vi "Reliability System MAIN (RT).vi"() -> ()   [LabVIEW 2013]
uses:
  TCP/PC/Event Mode.ctl
  RT subVIs/Controls/Stream RT FIFO Mode.ctl
  TCP/RT/RTsend PCrecv CMD.ctl
  <vilib>/FPGAPlugInAG/sbRIO-9626/niLvFpga_Open_sbRIO-9626.vi
  <vilib>/rvi/interface/common/dynamic/niFpgaDynamicAddResources.vi
  <vilib>/rvi/interface/common/niFpgaWaitOnOcc.vi
  <vilib>/Utility/error.llb/Error Cluster From Error Code.vi
  <vilib>/rvi/errors/niLvFpgaAdjustHostInterfaceError.vi
  <vilib>/Utility/file.llb/Read From Spreadsheet File (string).vi
  <vilib>/FPGAPlugInAG/Dynamic/niLvFpga_Reset_Dynamic.vi
  <vilib>/FPGAPlugInAG/Dynamic/niLvFpga_Run_Dynamic.vi
  <vilib>/rvi/interface/nirviOpenFPGA/nirviOpenFPGA.xnode
  FPGA Bitfiles/Reliability System.lvbitx
  FPGA/Reliability System (FPGA).vi
  <vilib>/rvi/interface/nirviMethod/nirviMethod.xnode
  <vilib>/rvi/interface/nirviReadWriteControl/nirviReadWriteControl.xnode
  <vilib>/NI_Real-Time Target Support.lvlib
  <vilib>/rvi/interface/Simulation/niFpgaSimulationCallBeginRW.vi
  NiFpgaLv.dll
  <vilib>/FPGAPlugInAG/Dynamic/niLvFpga_ReadFifo_Dynamic.vi
  <vilib>/rvi/errors/niLvFpgaMergeErrorWithErrorCode.vi
panel:
  out "Stream Error":i32
  out "FPGA Error":i32
  out "Sweeps Running":bool
  out "Sweep Count":i16
  out "Start  Ht Cmd":sgl
  out "End Ht Cmd":sgl
  out "Total Samples":sgl
  out "Start Sweep":bool
  out "Manual Cmd":bool
  out "Position Command Out":dbl
  out "Digital Output 4":bool
  out "Digital Output 3":bool
  out "Digital Output 2":bool
  out "Digital Output 1":bool
  out "Spare Output":dbl
  out "Power Supply Command":dbl
  out "Position Command":dbl
  in  "AI Loop Control (us)":u32
  in  "10kHz Loop Control (us)":u32
  in  "Stream Stop":bool
  out "RMC/DI7":bool
  out "RMC/DI6":bool
  out "RMC/DI5":bool
  out "RMC/DI4":bool
  out "AI Loop Time (us)":u32
  out "10kHz Loop Time (us)":u32
  out "Total (%)":dbl
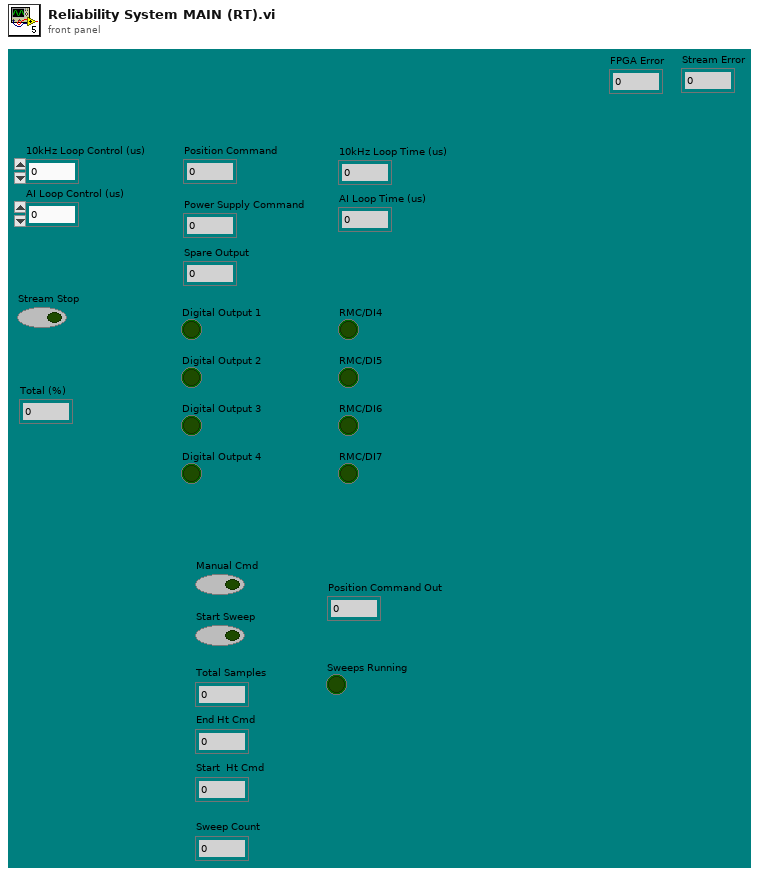
[diagram p1: front panel]
types:
  T1 = typedef "Event Mode.ctl" = enum16{"Init", "Get", "Set", "Destroy"}
  T2 = cluster{"DI Read Rate (sec)":dbl, "DI Read Timer":dbl, "Digital Outputs":bool[], "Analog Outputs":dbl[], "Sweeps Running":bool, "Sweep Parameters":sgl[], "Start Sweep":bool, "Manual Cmd":bool, "Startup Safety":bool, "Cal Cluster":cluster{"Slope":dbl[], "Offset":dbl[]}, "Cal Info":cluster{"Gauge#":i32, "CalDueDate":string}}
  T3 = enum16{"open", "replace", "create", "open or create", "replace or create", "replace or create with confirmation"}
  T4 = typedef "RTsend PCrecv CMD.ctl" = enum16{"Digital Inputs", "Connected?", "Data", "Data 2", "Cal2PC"}
  T5 = typedef "PCsend RTrecv CMD.ctl" = enum16{"ConnSettings", "Connect", "Stop", "Digital Outputs", "Analog Outputs", "Sweep Parameters", "Start Sweep", "Cal2RT", "Save Cal", "Load Cal"}
  T6 = cluster{"Slope":dbl[], "Offset":dbl[], "Gauge#":i32, "CalDueDate":string}
  T7 = cluster{"Sweeps Running":bool, dbl, "Current Sweep":i16}
  T8 = typedef "Stream RT FIFO Mode.ctl" = enum16{"Create", "Write", "Read", "Delete"}
  T9 = typedef "NI_Real-Time Target Support.lvlib/RT CPU Load.ctl" = cluster{"Total (%)":dbl, "Time Critical (%)":dbl, "Timed Structures (%)":dbl, "High (%)":dbl, "Above Normal (%)":dbl, "Normal (%)":dbl, "Background (%)":dbl, "Idle (%)":dbl, "ISR (%)":dbl}
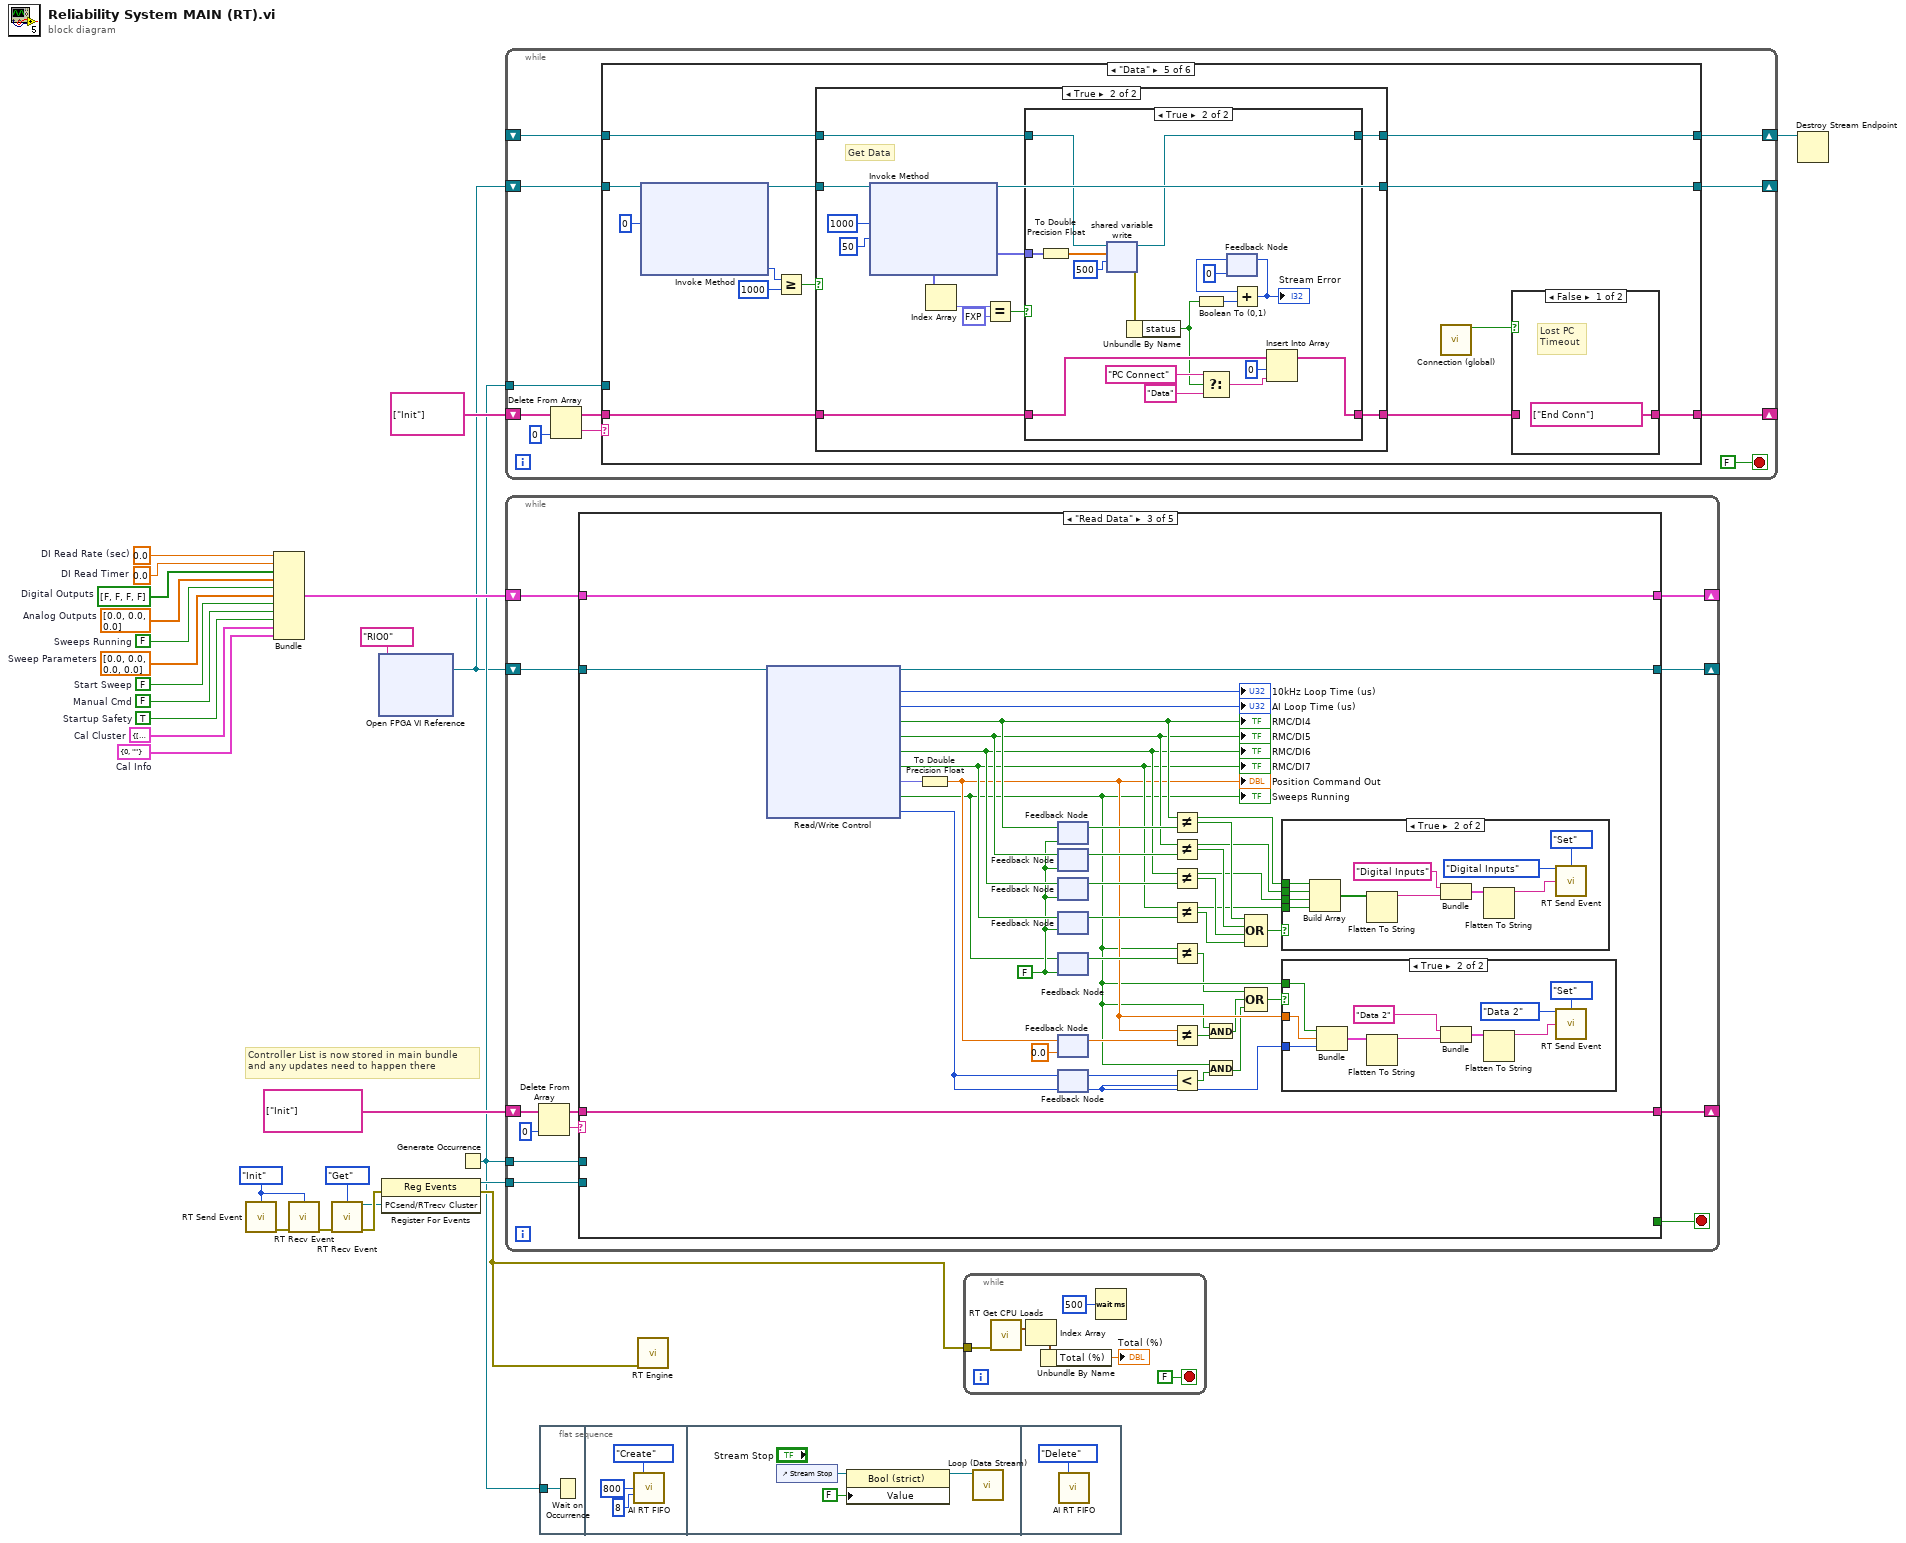
[diagram p0: block diagram]
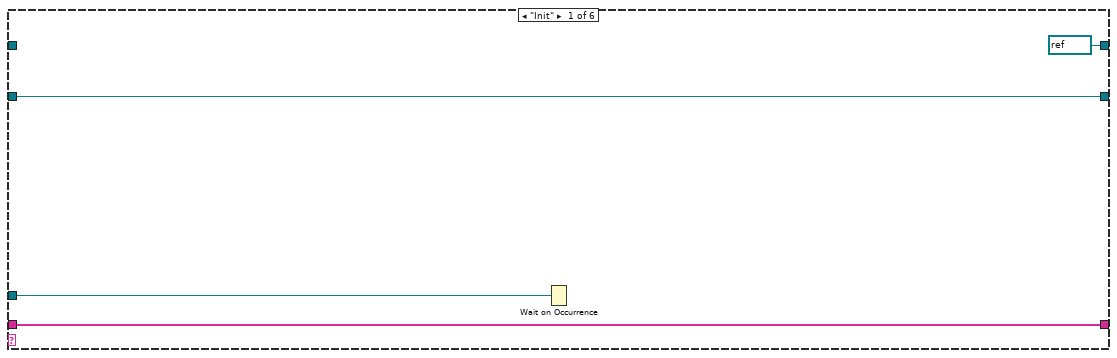
[diagram p2: hidden frame]
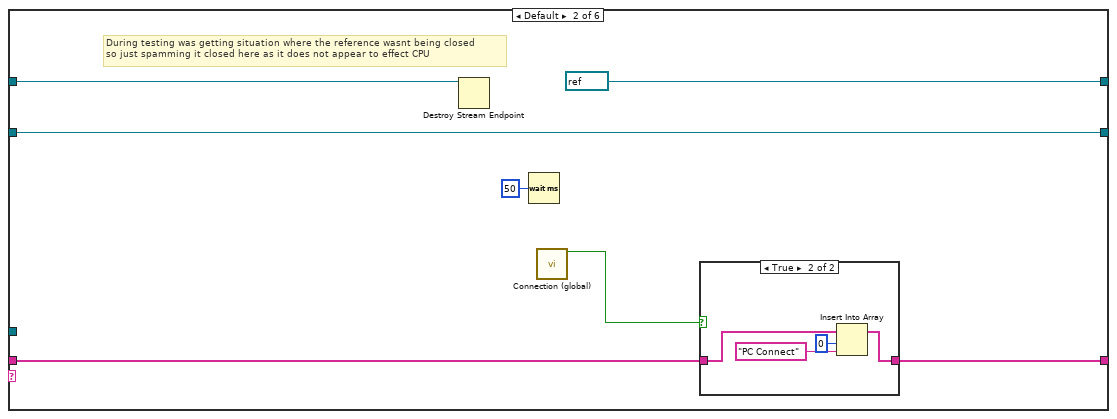
[diagram p3: hidden frame]
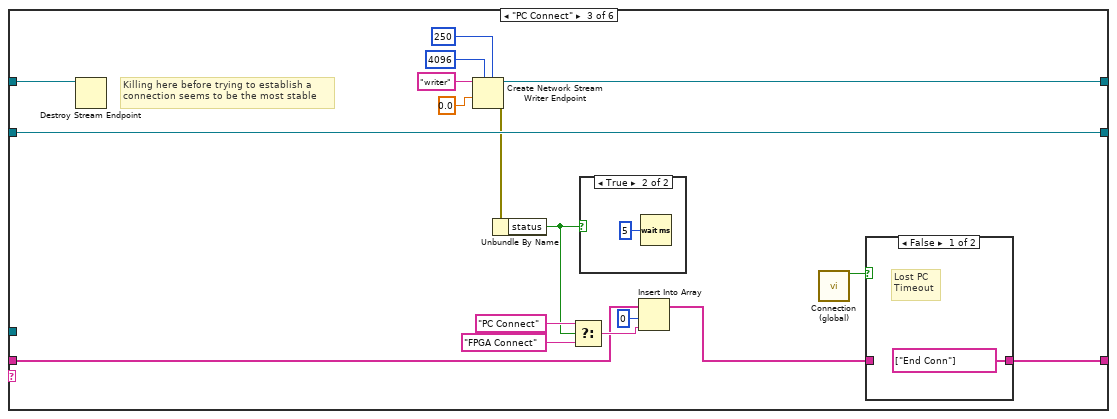
[diagram p5: hidden frame]
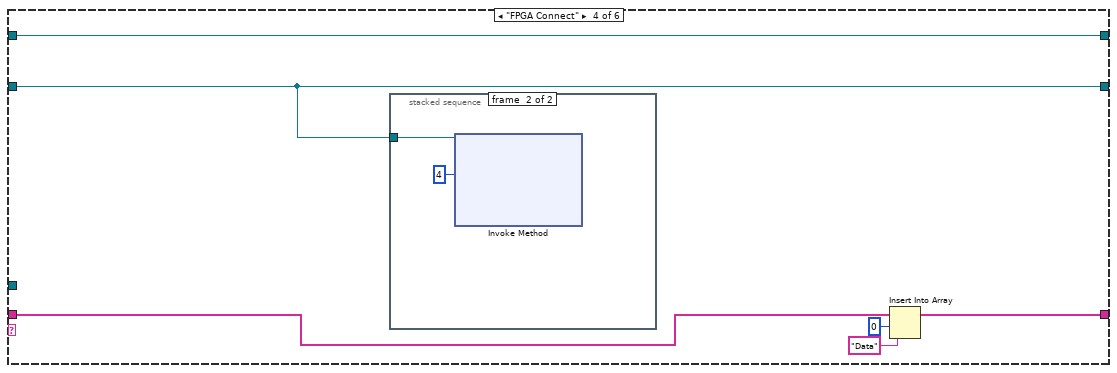
[diagram p8: hidden frame]
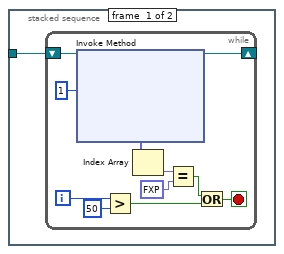
[diagram p9: hidden frame]
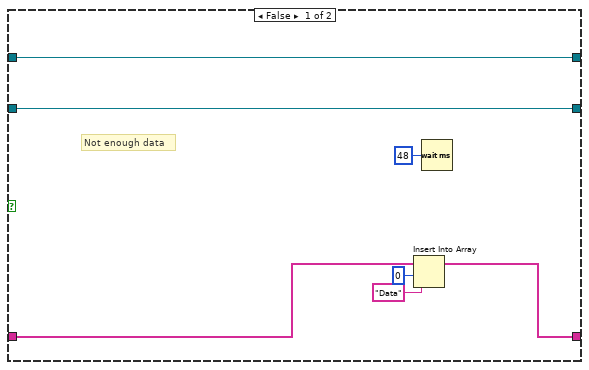
[diagram p11: hidden frame]
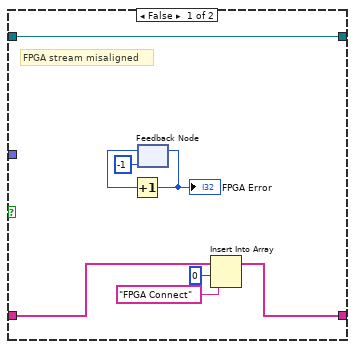
[diagram p12: hidden frame]
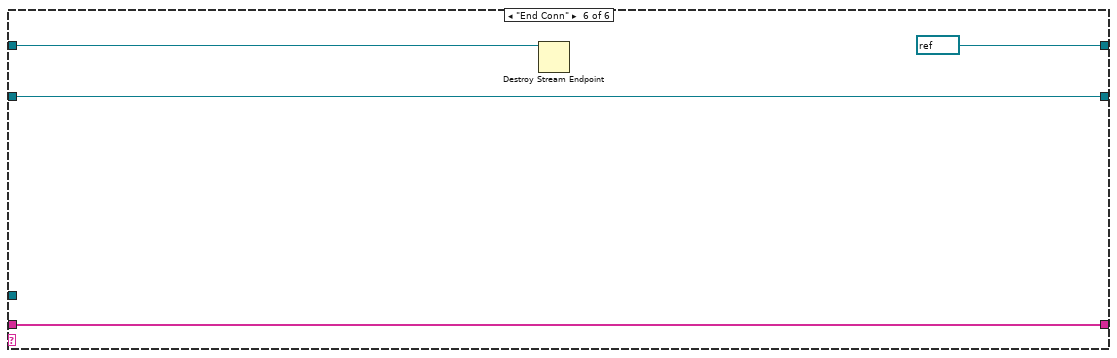
[diagram p13: hidden frame]
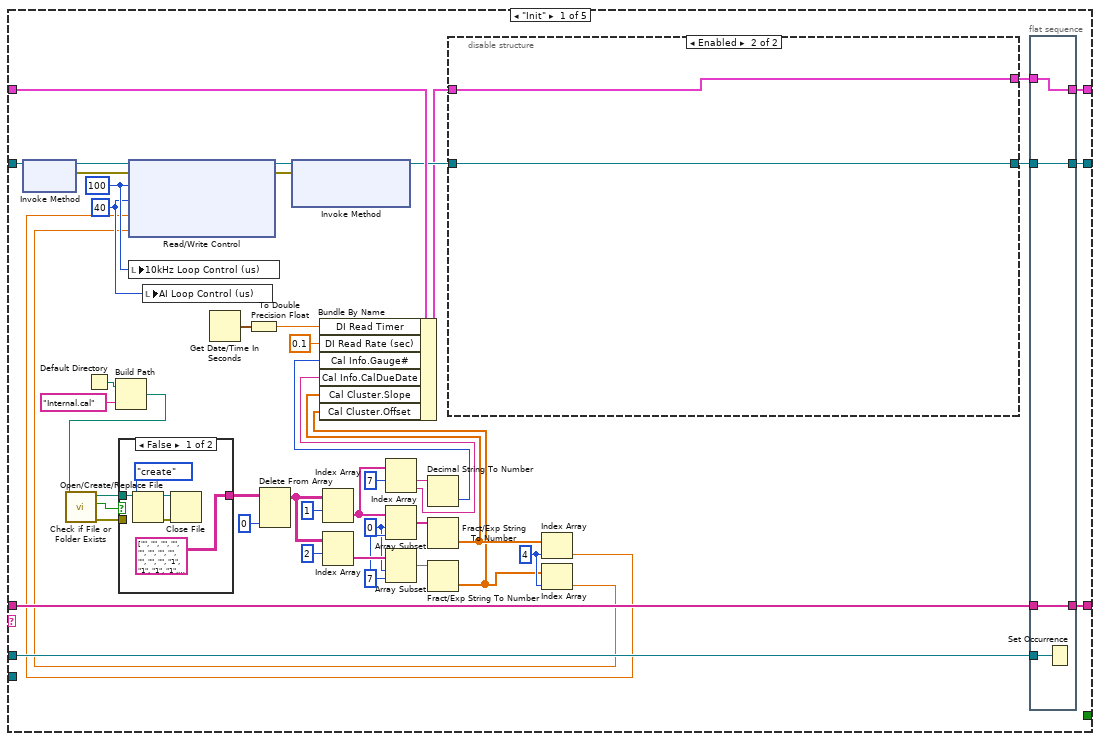
[diagram p14: hidden frame]
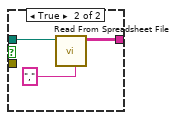
[diagram p15: hidden frame]
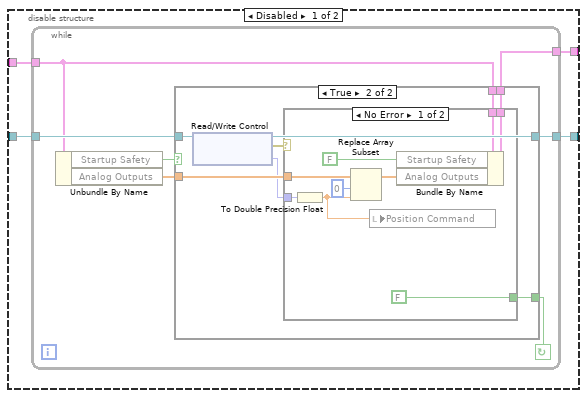
[diagram p16: hidden frame]
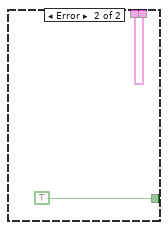
[diagram p18: hidden frame]
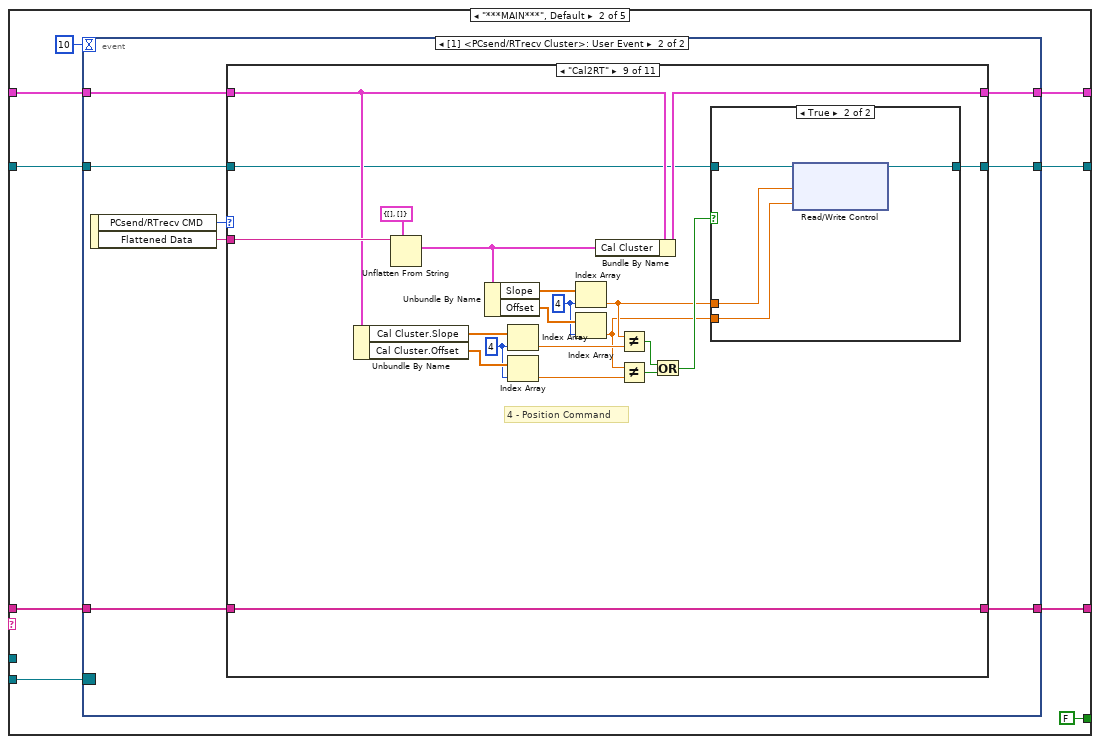
[diagram p19: hidden frame]
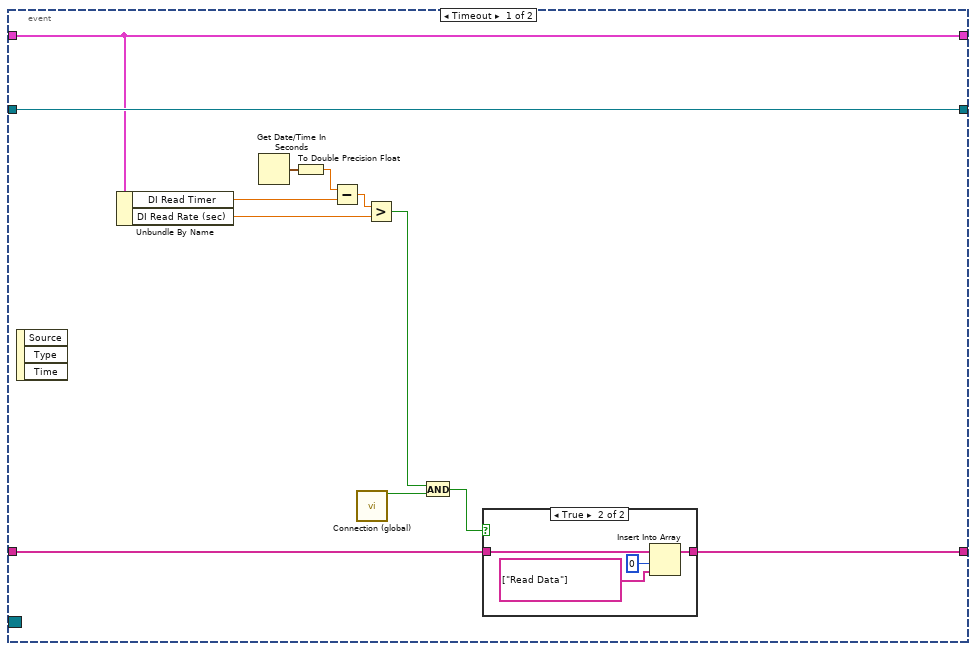
[diagram p20: hidden frame]
diagram:
  w3 = cluster{"Gauge#":i32, "CalDueDate":string} {"Gauge#"=0, "CalDueDate"=""}  # Cal Info
  w4 = cluster{"Slope":dbl[], "Offset":dbl[]} {"Slope"=[1.0, 1.0, 1.0, 1.0, 1.0, 1.0, 1.0], "Offset"=[0.0, 0.0, 0.0, 0.0, 0.0, 0.0, 0.0]}  # Cal Cluster
  w5 = TRUE  # Startup Safety
  w6 = FALSE  # Manual Cmd
  w7 = FALSE  # Start Sweep
  w8 = sgl[] [0.0, 0.0, 0.0, 0.0]  # Sweep Parameters
  w9 = FALSE  # Sweeps Running
  w12 = dbl[] [0.0, 0.0, 0.0]  # Analog Outputs
  w13 = bool[] [FALSE, FALSE, FALSE, FALSE]  # Digital Outputs
  w17 = 0.0  # DI Read Timer
  w18 = 0.0  # DI Read Rate (sec)
  w19 = Event_Mode."Init" ("Mode")
  # "Controller List is now stored in main bundle\nand any updates need to happen there"
  n1 = call "RT Send Event.vi"("Mode"=w19) -> ("Error Out"=w25:errorcluster)  [unwired: 13 in, 1 out]
  n2 = Bundle("DI Read Rate (sec)"=w18, "DI Read Timer"=w17, "Digital Outputs"=w13, "Analog Outputs"=w12, "Sweeps Running"=w9, "Sweep Parameters"=w8, "Start Sweep"=w7, "Manual Cmd"=w6, "Startup Safety"=w5, "Cal Cluster"=w4, "Cal Info"=w3) -> (w26:T2)  [unwired: 1 in]
  n3 = call "RT Recv Event.vi"("Mode"=w19, "Error In"=w25) -> ("Error Out"=w24:errorcluster)  [unwired: 12 in, 1 out]
  n4 = call "RT Recv Event.vi"("Mode"=Event_Mode."Get", "Error In"=w24) -> ("PCsend/RTrecv Cluster"=w22:refnum<user-event>, "Error Out"=w23:errorcluster)  [unwired: 12 in]
  n5 = xnode ("Open FPGA VI Reference")("resource name"=tag "RIO0") -> ("FPGA VI Reference Out"=w1:refnum<k20>)  [unwired: 1 in, 1 out]
  n6 = register-events(error in=w23, w22) -> (reference out=w21:refnum<event-registration>, error out=w16:errorcluster)  [unwired: 1 in]
  n7 = Generate Occurrence() -> (w10:refnum<k4>)
  n8 = while {
    shift-right: [w32] -> _
    shift-left: string[] ["Init"] -> [w36]
    tunnel: w10 -> [w31]
    shift-right: [w30] -> w2
    shift-left: _ -> [w29]
    shift-right: [w27] -> _
    shift-left: w1 -> [w28]
    stop <- FALSE stop-if-true
    n9 = Delete From Array(array=w36, index=0) -> (deleted portion=w34:string, array with subset deleted=w33:string[])  [unwired: 1 in]
    n10 = case shown="\"Data\"" w34 {
      tunnel: w33 -> [w40 w45 w64 w76 w97 w156]
      tunnel: [w40 w44 w57 w75 w95 w156] -> w32
      tunnel: w31 -> [w41 _ _ _ _ _]
      tunnel: [refnum<k21> refnum ("writer name") refnum<k21> refnum ("writer name") w55 w79 w98 refnum<k21> refnum ("writer name")] -> w30
      tunnel: w29 -> [_ w43 w54 w79 w99 w154]
      tunnel: w28 -> [w38 w48 w61 w78 w105 w155]
      tunnel: [w38 w48 w61 w78 w100 w155] -> w27
      frame "Init" {
        n11 = Wait on Occurrence(2:w41) -> ()  [unwired: 2 in, 1 out]
      }
      frame Default {
        # "During testing was getting situation where the reference wasnt being closed\nso just spamming it closed here as it does not appear to effect CPU"
        n12 = Destroy Stream Endpoint(11:w43) -> ()  [unwired: 1 in, 1 out]
        n13 = Wait (ms)(milliseconds to wait=u32 50) -> ()  [unwired: 1 out]
        n14 = call "Connection (global).vi"() -> ("PC Connected Out"=w46:bool)  [unwired: 15 in]
        n15 = case shown="True" w46 {
          tunnel: w45 -> [w49 w53]
          tunnel: [w49 w52] -> w44
          frame False {
          }
          frame True {
            n16 = Insert Into Array(array=w53, index=0, new element="PC Connect" ("new element/subarray")) -> (w52:string[])
          }
        }
      }
      frame "PC Connect" {
        # "Killing here before trying to establish a\nconnection seems to be the most stable"
        n17 = Destroy Stream Endpoint(11:w54) -> ()  [unwired: 1 in, 1 out]
        n18 = Create Network Stream Writer Endpoint(5:250 ("timeout in ms (-1)"), 7:4096 ("writer buffer size"), 9:0.0, 11:"writer" ("writer name")) -> (0:w56:errorcluster, 3:w55:refnum<k21>)  [unwired: 3 in]
        n19 = Unbundle By Name(w56) -> ("status"=w60:bool)
        n20 = Select(t="PC Connect" ("writer name"), s=w60, f="FPGA Connect" ("writer name")) -> (s? t:f=w66:string)
        n21 = case shown="True" w60 {
          frame False {
          }
          frame True {
            n22 = Wait (ms)(milliseconds to wait=u32 5) -> ()  [unwired: 1 out]
          }
        }
        n23 = Insert Into Array(array=w64, index=0, new element=w66) -> (w58:string[])
        n24 = call "Connection (global).vi"() -> ("PC Connected Out"=w59:bool)  [unwired: 15 in]
        n25 = case shown="False" w59 {
          tunnel: w58 -> [_ w72]
          tunnel: [string[] ["End Conn"] w72] -> w57
          frame False {
            # "Lost PC\nTimeout"
          }
          frame True {
            # "Still have PC\nContinue"
          }
        }
      }
      frame "FPGA Connect" {
        n26 = stacked-sequence {
          tunnel: w78 -> [w80 w93]
          frame #0 {
            n27 = while {
              shift-right: [w90] -> _
              shift-left: w80 -> [w91]
              i -> [w85]
              stop <- w82 stop-if-true
              n28 = xnode "Invoke Method"("FPGA VI Reference In"=w91, "Number of Elements"=u32 1) -> ("FPGA VI Reference Out"=w90:refnum<k20>, "Data"=w87:fxp<+/-,24,5>[])  [unwired: 2 in, 2 out]
              n29 = Greater?(x=w85, y=50) -> (0:w84:bool)
              n30 = Index Array(array=w87) -> (element=w86:fxp<+/-,24,5>)  [unwired: 1 in]
              n31 = Equal?(x=w86, y=fxp<+/-,24,5> -15.0) -> (x = y?=w83:bool)
              n32 = Or(x=w83, y=w84) -> (x .or. y?=w82:bool)
            }
          }
          frame #1 {
            n33 = xnode "Invoke Method"("FPGA VI Reference In"=w93, "Number of Elements"=u32 4) -> ()  [unwired: 2 in, 4 out]
          }
        }
        n34 = Insert Into Array(array=w76, index=0, new element="Data" ("new element/subarray")) -> (w75:string[])
      }
      frame "Data" {
        n35 = xnode "Invoke Method"("FPGA VI Reference In"=w105, "Number of Elements"=u32 0) -> ("FPGA VI Reference Out"=w101:refnum<k20>, "Elements Remaining"=w104:u32)  [unwired: 2 in, 2 out]
        n36 = Greater Or Equal?(x=w104, y=u32 1000) -> (x >= y?=w102:bool)
        n37 = case shown="True" w102 {
          tunnel: w101 -> [w114 w127]
          tunnel: [w114 w126] -> w100
          tunnel: w99 -> [w113 w120]
          tunnel: [w113 w119] -> w98
          tunnel: w97 -> [w112 w118]
          tunnel: [w111 w117] -> w96
          frame False {
            # "Not enough data"
            n38 = Insert Into Array(array=w112, index=0, new element="Data" ("new element/subarray")) -> (w111:string[])
            n39 = Wait (ms)(milliseconds to wait=u32 48) -> ()  [unwired: 1 out]
          }
          frame True {
            # "Get Data"
            n40 = xnode "Invoke Method"("FPGA VI Reference In"=w127, "Number of Elements"=u32 1000 ("y"), "Timeout (ms)"=50) -> ("FPGA VI Reference Out"=w126:refnum<k20>, "Data"=w116:fxp<+/-,24,5>[])  [unwired: 1 in, 2 out]
            n41 = Index Array(array=w116) -> (element=w122:fxp<+/-,24,5>)  [unwired: 1 in]
            n42 = Equal?(x=w122, y=fxp<+/-,24,5> -15.0) -> (x = y?=w121:bool)
            n43 = case shown="True" w121 {
              tunnel: w120 -> [w135 w151]
              tunnel: [w135 w150] -> w119
              tunnel: w118 -> [w134 w148]
              tunnel: [w131 w147] -> w117
              tunnel: w116 -> [_ w149]
              frame False {
                # "FPGA stream misaligned"
                n44 = feedback #1(-1) -> (w129:i32)
                n45 = Increment(x=w129) -> (x+1=w128:i32)
                "FPGA Error" <- w128
                n46 = feedback-in #1(w128) -> ()
                n47 = Insert Into Array(array=w134, index=0, new element="FPGA Connect" ("new element/subarray")) -> (w131:string[])
              }
              frame True {
                n48 = To Double Precision Float(number=w149) -> (double precision float=w141:dbl[])
                n49 = shared-variable-write(w151, w141, 500 ("timeout ms (-1)")) -> (w150:refnum<k21>, w145:errorcluster)  [unwired: 1 in, 1 out]
                n50 = Unbundle By Name(w145) -> ("status"=w136:bool)
                n51 = Boolean To (0,1)(Boolean=w136) -> (0, 1=w137:i16)
                n52 = Select(t="PC Connect", s=w136, f="Data") -> (s? t:f=w142:string)
                n53 = feedback #2(0) -> (w139:i32)
                n54 = Add(x=w139, y=w137) -> (x+y=w138:i32)
                "Stream Error" <- w138
                n55 = feedback-in #2(w138) -> ()
                n56 = Insert Into Array(array=w148, index=0, new element=w142) -> (w147:string[])
              }
            }
          }
        }
        n57 = call "Connection (global).vi"() -> ("PC Connected Out"=w94:bool)  [unwired: 15 in]
        n58 = case shown="False" w94 {
          tunnel: w96 -> [_ w108]
          tunnel: [string[] ["End Conn"] w108] -> w95
          frame False {
            # "Lost PC\nTimeout"
          }
          frame True {
            # "Still have PC\nContinue"
          }
        }
      }
      frame "End Conn" {
        n59 = Destroy Stream Endpoint(11:w154) -> ()  [unwired: 1 in, 1 out]
      }
    }
  }
  n60 = while {
    shift-right: [w164] -> _
    shift-left: string[] ["Init"] -> [w168]
    shift-right: [w161] -> _
    shift-left: w26 -> [w163]
    shift-right: [w159] -> _
    shift-left: w1 -> [w160]
    tunnel: w21 -> [w158]
    tunnel: w10 -> [w157]
    stop <- w162 stop-if-true
    n61 = Delete From Array(array=w168, index=0) -> (deleted portion=w165:string, array with subset deleted=w166:string[])  [unwired: 1 in]
    n62 = case shown="\"Read Data\"" w165 {
      tunnel: w166 -> [w211 w270 w476 w523 w590]
      tunnel: [w210 w266 w476 w523 w589] -> w164
      tunnel: w163 -> [w207 w269 w459 w503 w595]
      tunnel: [_ FALSE _ _ _] -> w162
      tunnel: [w196 w267 w459 w502 w594] -> w161
      tunnel: w160 -> [w213 w264 w477 w505 w597]
      tunnel: [w212 w263 w475 w522 w597] -> w159
      tunnel: w158 -> [_ w262 _ _ _]
      tunnel: w157 -> [w209 _ _ _ _]
      frame "Init" {
        w173 = 4 ("index")
        w187 = 7 ("length")
        w186 = 0 ("index")
        w178 = u32 40 ("100kHz Loop Control (us)")
        w201 = u32 100 ("10kHz Loop Control (us)")
        n63 = xnode "Invoke Method"("FPGA VI Reference In"=w213) -> ("FPGA VI Reference Out"=w206:refnum<k20>, "error out"=w205:errorcluster)  [unwired: 1 in]
        n64 = Default Directory() -> (w176:path)
        n65 = Build Path(base path=w176, name or relative path="Internal.cal") -> (appended path=w174:path)
        n66 = call <vilib>:"Check if File or Folder Exists.vi"("path"=w174) -> ("error out"=w177:errorcluster, "file or folder exists?"=w194:bool, "dup path"=w195:path)  [unwired: 8 in]
        n67 = case shown="False" w194 {
          tunnel: [string[][] [["", "", "", "", "", "", "", "", "", ""], ["", "1", "1", "1", "1", "1", "1", "1", "1234", "01/01/00"], ["", "0", "0", "0", "0", "0", "0", "0", "0", "0"]] ("all rows") w222] -> w185
          tunnel: w195 -> [w219 w220]
          tunnel: w177 -> [_ _]
          frame False {
            n68 = Open/Create/Replace File(file path (use dialog)=w219, operation (0:open)=T3."create") -> (refnum out=w218:refnum<file>, error out=w217:errorcluster)  [unwired: 4 in, 1 out]
            n69 = Close File(refnum=w218, error in=w217) -> ()  [unwired: 2 out]
          }
          frame True {
            n70 = call-poly <vilib>:"Read From Spreadsheet File.vi"("delimiter (\\t)"="," ("delimiter (\\t)"), "file path (dialog if empty)"=w220) -> ("all rows"=w222:string[][])  [unwired: 5 in, 4 out]
          }
        }
        n71 = local write "10kHz Loop Control (us)"(w201) -> ()
        n72 = local write "AI Loop Control (us)"(w178) -> ()
        n73 = Get Date/Time In Seconds() -> (seconds since 1Jan1904=w214:timestamp)
        n74 = To Double Precision Float(number=w214) -> (double precision float=w208:dbl)
        n75 = Delete From Array(array=w185, index (col)=0 ("disabled index (col)")) -> (array with subset deleted=w183:string[][])  [unwired: 2 in, 1 out]
        n76 = Index Array(array=w183, index (row)=1) -> (element=w191:string[])  [unwired: 1 in]
        n77 = Index Array(array=w183, index (row)=2) -> (element=w188:string[])  [unwired: 1 in]
        n78 = Index Array(array=w191, index #1=7 ("index")) -> (element #1=w193:string, element #2=w179:string)  [unwired: 1 in]
        n79 = Array Subset(array=w191, index=w186, length=w187) -> (w189:string[])
        n80 = Array Subset(array=w188, index=w186, length=w187) -> (w190:string[])
        n81 = Decimal String To Number(string=w193) -> (number=w180:i32)  [unwired: 2 in, 1 out]
        n82 = Fract/Exp String To Number(string=w189) -> (number=w172:dbl[])  [unwired: 3 in, 1 out]
        n83 = Fract/Exp String To Number(string=w190) -> (number=w171:dbl[])  [unwired: 3 in, 1 out]
        n84 = Bundle By Name(cluster=w207, "DI Read Timer"=w208, "DI Read Rate (sec)"=0.1, "Cal Info.Gauge#"=w180, "Cal Info.CalDueDate"=w179, "Cal Cluster.Slope"=w172, "Cal Cluster.Offset"=w171) -> (w198:T2)
        n85 = Index Array(array=w172, index=w173) -> (element=w170:dbl)
        n86 = Index Array(array=w171, index=w173) -> (element=w169:dbl)
        n87 = xnode "Read/Write Control"("FPGA VI Reference In"=w206, "error in"=w205, "10kHz Loop Control (us)"=w201, "AI Loop Control (us)"=w178, "Ht Cmd Slope"=w170, "Ht Cmd Offset"=w169) -> ("FPGA VI Reference Out"=w203:refnum<k20>, "error out"=w204:errorcluster)
        n88 = xnode "Invoke Method"("FPGA VI Reference In"=w203, "error in"=w204) -> ("FPGA VI Reference Out"=w200:refnum<k20>)  [unwired: 1 in, 1 out]
        n89 = disable-structure shown="Enabled" {
          disable-tunnel: w200 -> [w226 w256]
          disable-tunnel: [w225 w256] -> w199
          disable-tunnel: w198 -> [w224 w257]
          disable-tunnel: [w223 w257] -> w197
          frame Disabled {
            n90 = while {
              tunnel: w226 -> [w231]
              tunnel: [w230] -> w225
              tunnel: w224 -> [w229]
              tunnel: [w228] -> w223
              stop <- w227 continue-if-true
              n91 = Unbundle By Name(w229) -> ("Startup Safety"=w233:bool, "Analog Outputs"=w232:dbl[])
              n92 = case shown="True" w233 {
                selector: w233 -> [w234 _]
                tunnel: w231 -> [w236 w244]
                tunnel: [w236 w243] -> w230
                tunnel: [w235 w241] -> w228
                tunnel: w229 -> [w235 w240]
                tunnel: w232 -> [_ w239]
                tunnel: [w234 w237] -> w227
                frame False {
                }
                frame True {
                  n93 = xnode "Read/Write Control"("FPGA VI Reference In"=w244) -> ("FPGA VI Reference Out"=w243:refnum<k20>, "error out"=w242:errorcluster, "Height Raw"=w238:fxp<+/-,24,5>)  [unwired: 1 in]
                  n94 = case shown="No Error" w242 {
                    tunnel: [w253 w255] -> w241
                    tunnel: w240 -> [w252 w255]
                    tunnel: w239 -> [w251 _]
                    tunnel: w238 -> [w248 _]
                    tunnel: [FALSE TRUE] -> w237
                    frame No Error {
                      n95 = To Double Precision Float(number=w248) -> (double precision float=w247:dbl)
                      n96 = Replace Array Subset(array=w251, new element=w247, index=0) -> (w250:dbl[])
                      n97 = local write "Position Command"(w247) -> ()
                      n98 = Bundle By Name(cluster=w252, "Startup Safety"=FALSE, "Analog Outputs"=w250) -> (w253:T2)
                    }
                    frame Error {
                    }
                  }
                }
              }
            }
          }
          frame Enabled {
          }
        }
        n99 = flat-sequence {
          tunnel: [w259] -> w212
          tunnel: w211 -> [w261]
          tunnel: [w261] -> w210
          tunnel: w209 -> [w260]
          tunnel: w199 -> [w259]
          tunnel: w197 -> [w258]
          tunnel: [w258] -> w196
          frame #0 {
            n100 = Set Occurrence(w260) -> ()
          }
        }
      }
      frame "***MAIN***", Default {
        n101 = event shown="[1] <PCsend/RTrecv Cluster>: User Event" {
          selector: w262 -> [_ _]
          dyn-events: _ -> [_ _]
          timeout: 10 -> [_ _]
          tunnel: w270 -> [w280 w292]
          tunnel: w269 -> [w274 w295]
          tunnel: [w274 w294] -> w267
          tunnel: [w275 w291] -> w266
          tunnel: w264 -> [w279 w288]
          tunnel: [w279 w290] -> w263
          event Timeout {
            n102 = event-data() -> ()  [unwired: 1 in, 3 out]
            n103 = Unbundle By Name(w274) -> ("DI Read Timer"=w282:dbl, "DI Read Rate (sec)"=w281:dbl)
            n104 = Get Date/Time In Seconds() -> (seconds since 1Jan1904=w278:timestamp)
            n105 = To Double Precision Float(number=w278) -> (double precision float=w276:dbl)
            n106 = Subtract(x=w276, y=w282) -> (x-y=w277:dbl)
            n107 = call "Connection (global).vi"() -> ("PC Connected Out"=w273:bool)  [unwired: 15 in]
            n108 = Greater?(x=w277, y=w281) -> (0:w272:bool)
            n109 = And(x=w272, y=w273) -> (x .and. y?=w271:bool)
            n110 = case shown="True" w271 {
              tunnel: w280 -> [w283 w287]
              tunnel: [w283 w286] -> w275
              frame False {
              }
              frame True {
                n111 = Insert Into Array(array=w287, index=0, new element=string[] ["Read Data"]) -> (w286:string[])
              }
            }
          }
          event User Event {
            n112 = event-data() -> ("PCsend/RTrecv CMD"=w289:T5, "Flattened Data"=w293:string)  [unwired: 1 in]
            n113 = case shown="\"Cal2RT\"" w289 {
              tunnel: w295 -> [w298 w300 w303 w306 w315 w328 w348 w365 w385 w427 w434]
              tunnel: [w298 w300 w303 w306 w314 w322 w347 w363 w386 w428 w434] -> w294
              tunnel: w293 -> [_ _ _ _ w321 w337 w350 w366 w387 w429 _]
              tunnel: w292 -> [w297 w299 w302 w305 w319 w333 w344 w360 w372 w426 w443]
              tunnel: [w297 w299 w302 w305 w318 w332 w344 w359 w372 w426 w443] -> w291
              tunnel: w288 -> [w296 w301 w304 w307 w313 w338 w346 w362 w370 w425 w442]
              tunnel: [w296 w301 w304 w307 w313 w338 w346 w362 w369 w425 w442] -> w290
              frame Default {
                # "Shouldn't ever get here\nwhich would mean something is not setup correctly"
              }
              frame "ConnSettings" {
              }
              frame "Connect" {
              }
              frame "Stop" {
              }
              frame "Digital Outputs" {
                n114 = Unflatten From String(type=bool[] [FALSE, FALSE, FALSE, FALSE], binary string=w321) -> (value=w312:bool[])  [unwired: 3 in, 2 out]
                n115 = Index Array(array=w312) -> (element #1=→"Digital Output 1":bool, element #2=→"Digital Output 2":bool, element #3=→"Digital Output 3":bool, element #4=→"Digital Output 4":bool)  [unwired: 4 in]
                n116 = Bundle By Name(cluster=w315, "Digital Outputs"=w312) -> (w314:T2)
                n117 = Insert Into Array(array=w319, index=0, new element="Write Outputs" ("new element/subarray")) -> (w318:string[])
              }
              frame "Analog Outputs" {
                n118 = Unflatten From String(type=dbl[] [0.0, 0.0, 0.0], binary string=w337) -> (value=w331:dbl[])  [unwired: 3 in, 2 out]
                n119 = Unbundle By Name(w328) -> ("Analog Outputs"=w327:dbl[])
                n120 = Index Array(array=w331) -> (element #1=w325:dbl, element #2=→"Power Supply Command":dbl, element #3=→"Spare Output":dbl)  [unwired: 3 in]
                "Position Command" <- w325
                n121 = Index Array(array=w327) -> (element=w326:dbl)  [unwired: 1 in]
                n122 = Bundle By Name(cluster=w328, "Analog Outputs"=w331) -> (w323:T2)
                n123 = Not Equal?(x=w326, y=w325) -> (x != y?=w324:bool)
                n124 = Insert Into Array(array=w333, index=0, new element="Write Outputs" ("new element/subarray")) -> (w332:string[])
                n125 = case shown="True" w324 {
                  tunnel: w323 -> [w339 w343]
                  tunnel: [w339 w341] -> w322
                  frame False {
                  }
                  frame True {
                    w340 = TRUE ("Manual Cmd")
                    n126 = local write "Manual Cmd"(w340) -> ()
                    n127 = Bundle By Name(cluster=w343, "Manual Cmd"=w340, "Start Sweep"=FALSE) -> (w341:T2)
                  }
                }
              }
              frame "Sweep Parameters" {
                n128 = Unflatten From String(type=sgl[] [0.0, 0.0, 0.0, 0.0], binary string=w350) -> (value=w345:sgl[])  [unwired: 3 in, 2 out]
                n129 = Index Array(array=w345) -> (element #1=→"Total Samples":sgl, element #2=→"End Ht Cmd":sgl, element #3=→"Start  Ht Cmd":sgl, element #4=w354:sgl)  [unwired: 4 in]
                n130 = To Word Integer(number=w354) -> (16bit integer=→"Sweep Count":i16)
                n131 = Bundle By Name(cluster=w348, "Sweep Parameters"=w345) -> (w347:T2)
              }
              frame "Start Sweep" {
                n132 = Unflatten From String(type=FALSE, binary string=w366) -> (value=w357:bool)  [unwired: 3 in, 2 out]
                "Start Sweep" <- w357
                n133 = Not(x=w357) -> (.not. x?=w356:bool)
                "Manual Cmd" <- w356
                n134 = Insert Into Array(array=w360, index=0, new element=string[] ["Write Outputs", "Handle Sweep Start"]) -> (w359:string[])
                n135 = Bundle By Name(cluster=w365, "Start Sweep"=w357, "Manual Cmd"=w356) -> (w363:T2)
              }
              frame "Cal2RT" {
                w378 = 4 ("index")
                w377 = 4 ("index")
                # "4 - Position Command"
                n136 = Unbundle By Name(w385) -> ("Cal Cluster.Slope"=w382:dbl[], "Cal Cluster.Offset"=w381:dbl[])
                n137 = Unflatten From String(type=cluster{"Slope":dbl[], "Offset":dbl[]} {"Slope"=[], "Offset"=[]}, binary string=w387) -> (value=w383:cluster{"Slope":dbl[], "Offset":dbl[]})  [unwired: 3 in, 2 out]
                n138 = Unbundle By Name(w383) -> ("Slope"=w380:dbl[], "Offset"=w379:dbl[])
                n139 = Index Array(array=w382, index=w377) -> (element=w376:dbl)
                n140 = Index Array(array=w381, index=w377) -> (element=w375:dbl)
                n141 = Index Array(array=w380, index=w378) -> (element=w368:dbl)
                n142 = Index Array(array=w379, index=w378) -> (element=w367:dbl)
                n143 = Bundle By Name(cluster=w385, "Cal Cluster"=w383) -> (w386:T2)
                n144 = Not Equal?(x=w368, y=w376) -> (x != y?=w374:bool)
                n145 = Not Equal?(x=w367, y=w375) -> (x != y?=w373:bool)
                n146 = Or(x=w374, y=w373) -> (x .or. y?=w371:bool)
                n147 = case shown="True" w371 {
                  tunnel: w370 -> [w388 w392]
                  tunnel: [w388 w391] -> w369
                  tunnel: w368 -> [_ w390]
                  tunnel: w367 -> [_ w389]
                  frame False {
                  }
                  frame True {
                    n148 = xnode "Read/Write Control"("FPGA VI Reference In"=w392, "Ht Cmd Slope"=w390, "Ht Cmd Offset"=w389) -> ("FPGA VI Reference Out"=w391:refnum<k20>)  [unwired: 1 in, 1 out]
                  }
                }
              }
              frame "Save Cal" {
                (unwired) path "c/Internal.cal"
                w402 = ""
                n149 = Unbundle By Name(w427) -> ("Cal Cluster.Slope"=w399:dbl[], "Cal Cluster.Offset"=w396:dbl[])
                n150 = Unflatten From String(type=cluster{"Gauge#":i32, "CalDueDate":string} {"Gauge#"=0, "CalDueDate"=""}, binary string=w429) -> (value=w400:cluster{"Gauge#":i32, "CalDueDate":string})  [unwired: 3 in, 2 out]
                n151 = Unbundle By Name(w400) -> ("Gauge#"=w398:i32, "CalDueDate"=w397:string)
                n152 = Default Directory() -> (w395:path)
                n153 = Number To Decimal String(number=w398) -> (decimal integer string=w401:string)  [unwired: 1 in]
                n154 = Number To Fractional String(number=w399) -> (F-format string=w406:string[])  [unwired: 3 in]
                n155 = Number To Fractional String(number=w396) -> (F-format string=w404:string[])  [unwired: 3 in]
                n156 = Build Path(base path=w395, name or relative path="Internal.cal") -> (appended path=w393:path)
                n157 = Build Array (concatenate)(w406, w401, w397) -> (w405:string[])
                n158 = Build Array (concatenate)(w404, w402, w402) -> (w403:string[])
                n159 = Replace Array Subset(array=string[][] [["Power Supply Voltage", "Level Sender Voltage", "AI-3 Spare", "Height Gauge", "Servo Motor Control", "Spare Analog Output 1", "Spare Analog Output 2", "Gauge Number", "CalDueDate"], ["", "", "", "", "", "", "", "", ""], ["", "", "", "", "", "", "", "", ""]], new element=w405, index (row)=1) -> (w414:string[][])  [unwired: 1 in]
                n160 = Bundle By Name(cluster=w427, "Cal Info"=w400) -> (w428:T2)
                n161 = Replace Array Subset(array=w414, new element=w403, index (row)=2) -> (w413:string[][])  [unwired: 1 in]
                n162 = Insert Into Array(array=w413, index (col)=0 ("disabled index (col)"), new element=string[] ["Channel Name", "Slope", "Offset"]) -> (w408:string[][])  [unwired: 1 in]
                n163 = Open/Create/Replace File(file path (use dialog)=w393, operation (0:open)=T3."open or create") -> (refnum out=w416:refnum<file>, error out=w415:errorcluster)  [unwired: 4 in, 1 out]
                n164 = Array To Spreadsheet String(delimiter (Tab)=",", array=w408, 3:"%s" ("format string")) -> (spreadsheet string=w418:string)
                n165 = Write to Text File(file (use dialog)=w416, text=w418, error in=w415) -> (refnum out=w422:refnum<file>, error out=w423:errorcluster)  [unwired: 1 in, 1 out]
                n166 = Close File(refnum=w422, error in=w423) -> (error out=w421:errorcluster)  [unwired: 1 out]
                n167 = call <vilib>:"Clear Errors.vi"("error in (no error)"=w421) -> ()  [unwired: 6 in, 1 out]
              }
              frame "Load Cal" {
                # "This is a request from the PC to be sent the cal file settings"
                n168 = Unbundle By Name(w434) -> ("Cal Cluster.Slope"=w433:dbl[], "Cal Cluster.Offset"=w432:dbl[], "Cal Info.Gauge#"=w431:i32, "Cal Info.CalDueDate"=w430:string)
                n169 = Bundle("Slope"=w433, "Offset"=w432, "Gauge#"=w431, "CalDueDate"=w430) -> (w436:T6)  [unwired: 1 in]
                n170 = Flatten To String(anything=w436) -> (data string=w440:string)  [unwired: 3 in, 2 out]
                n171 = Bundle("Cal2PC", "data string"=w440) -> (w439:cluster{string, "data string":string})  [unwired: 1 in]
                n172 = Flatten To String(anything=w439) -> (data string=w437:string)  [unwired: 3 in, 2 out]
                n173 = call "RT Send Event.vi"("RTsend/PCrecv CMD"=RTsend_PCrecv_CMD."Cal2PC", "Mode"=Event_Mode."Set", "Flattened Data"=w437) -> ()  [unwired: 11 in, 2 out]
              }
            }
          }
        }
      }
      frame "Read Data" {
        w458 = FALSE ("RMC/DI7")
        n174 = xnode "Read/Write Control"("FPGA VI Reference In"=w477) -> ("FPGA VI Reference Out"=w475:refnum<k20>, "10kHz Loop Time (us)"=→"10kHz Loop Time (us)":u32, "AI Loop Time (us)"=→"AI Loop Time (us)":u32, "RMC/DI4"=w465:bool, "RMC/DI5"=w464:bool, "RMC/DI6"=w463:bool, "RMC/DI7"=w462:bool, "Position Cmd Out"=w455:fxp<+/-,27,12>, "Sweeps Running"=w452:bool, "Current Sweep"=w446:i16)  [unwired: 1 in, 1 out]
        "RMC/DI4" <- w465
        "RMC/DI5" <- w464
        "RMC/DI6" <- w463
        "RMC/DI7" <- w462
        "Sweeps Running" <- w452
        n175 = To Double Precision Float(number=w455) -> (double precision float=w454:dbl)
        "Position Command Out" <- w454
        n176 = feedback-in #3(w465) -> ()
        n177 = feedback #3(w458) -> (w473:bool)
        n178 = feedback #4(w458) -> (w472:bool)
        n179 = feedback-in #4(w464) -> ()
        n180 = feedback #5(w458) -> (w471:bool)
        n181 = feedback-in #5(w463) -> ()
        n182 = feedback #6(w458) -> (w470:bool)
        n183 = feedback-in #6(w462) -> ()
        n184 = feedback #7(w458) -> (w457:bool)
        n185 = feedback-in #7(w452) -> ()
        n186 = feedback #8(0.0) -> (w460:dbl)
        n187 = feedback-in #8(w454) -> ()
        n188 = feedback #9(w446) -> (w453:i16)
        n189 = feedback-in #9(w446) -> ()
        n190 = Not Equal?(x=w465, y=w473) -> (x != y?=w469:bool)
        n191 = Not Equal?(x=w464, y=w472) -> (x != y?=w468:bool)
        n192 = Not Equal?(x=w463, y=w471) -> (x != y?=w467:bool)
        n193 = Not Equal?(x=w462, y=w470) -> (x != y?=w466:bool)
        n194 = Not Equal?(x=w452, y=w457) -> (x != y?=w450:bool)
        n195 = Not Equal?(x=w454, y=w460) -> (x != y?=w456:bool)
        n196 = Less?(x=w453, y=w446) -> (x < y?=w451:bool)
        n197 = And(x=w452, y=w456) -> (x .and. y?=w448:bool)
        n198 = And(x=w452, y=w451) -> (x .and. y?=w447:bool)
        n199 = Compound Arithmetic op=OR(w469, w468, w467, w466) -> (w474:bool)
        n200 = Compound Arithmetic op=OR(w450, w448, w447) -> (w449:bool)
        n201 = case shown="True" w474 {
          tunnel: w462 -> [_ w496]
          tunnel: w463 -> [_ w495]
          tunnel: w464 -> [_ w494]
          tunnel: w465 -> [_ w493]
          frame False {
          }
          frame True {
            n202 = Build Array(w493, w494, w495, w496) -> (w492:bool[])
            n203 = Flatten To String(anything=w492) -> (data string=w491:string)  [unwired: 3 in, 2 out]
            n204 = Bundle("Digital Inputs", "data string"=w491) -> (w490:cluster{string, "data string":string})  [unwired: 1 in]
            n205 = Flatten To String(anything=w490) -> (data string=w488:string)  [unwired: 3 in, 2 out]
            n206 = call "RT Send Event.vi"("RTsend/PCrecv CMD"=RTsend_PCrecv_CMD."Digital Inputs", "Mode"=Event_Mode."Set", "Flattened Data"=w488) -> ()  [unwired: 11 in, 2 out]
          }
        }
        n207 = case shown="True" w449 {
          tunnel: w452 -> [_ w482]
          tunnel: w454 -> [_ w481]
          tunnel: w446 -> [_ w478]
          frame False {
          }
          frame True {
            n208 = Bundle("Sweeps Running"=w482, w481, "Current Sweep"=w478) -> (w480:T7)  [unwired: 1 in]
            n209 = Flatten To String(anything=w480) -> (data string=w486:string)  [unwired: 3 in, 2 out]
            n210 = Bundle("Data 2", "data string"=w486) -> (w485:cluster{string, "data string":string})  [unwired: 1 in]
            n211 = Flatten To String(anything=w485) -> (data string=w483:string)  [unwired: 3 in, 2 out]
            n212 = call "RT Send Event.vi"("RTsend/PCrecv CMD"=RTsend_PCrecv_CMD."Data 2", "Mode"=Event_Mode."Set", "Flattened Data"=w483) -> ()  [unwired: 11 in, 2 out]
          }
        }
      }
      frame "Write Outputs" {
        # "#Change"
        # "Prevent movement on initialization"
        n213 = disable-structure shown="Disabled" {
          disable-tunnel: w505 -> [w529 w554]
          disable-tunnel: [w528 w554] -> w504
          disable-tunnel: w503 -> [w527 w555]
          disable-tunnel: [w526 w555] -> w502
          disable-tunnel: [w524 FALSE] -> w501
          frame Disabled {
            n214 = Unbundle By Name(w527) -> ("Startup Safety"=w530:bool, "Analog Outputs"=w525:dbl[])
            n215 = case shown="True" w530 {
              selector: w530 -> [w531 _]
              tunnel: w529 -> [w533 w541]
              tunnel: [w533 w540] -> w528
              tunnel: [w532 w538] -> w526
              tunnel: w527 -> [w532 w537]
              tunnel: w525 -> [_ w536]
              tunnel: [w531 w534] -> w524
              frame False {
              }
              frame True {
                n216 = xnode "Read/Write Control"("FPGA VI Reference In"=w541) -> ("FPGA VI Reference Out"=w540:refnum<k20>, "error out"=w539:errorcluster, "Height Raw"=w535:fxp<+/-,24,5>)  [unwired: 1 in]
                n217 = case shown="No Error" w539 {
                  tunnel: [w550 w552] -> w538
                  tunnel: w537 -> [w549 w552]
                  tunnel: w536 -> [w548 _]
                  tunnel: w535 -> [w545 _]
                  tunnel: [FALSE TRUE] -> w534
                  frame No Error {
                    n218 = To Double Precision Float(number=w545) -> (double precision float=w544:dbl)
                    n219 = Replace Array Subset(array=w548, new element=w544, index=0) -> (w547:dbl[])
                    n220 = local write "Position Command"(w544) -> ()
                    n221 = Bundle By Name(cluster=w549, "Startup Safety"=FALSE, "Analog Outputs"=w547) -> (w550:T2)
                  }
                  frame Error {
                  }
                }
              }
            }
          }
          frame Enabled {
          }
        }
        n222 = Unbundle By Name(w502) -> ("Digital Outputs"=w515:bool[], "Analog Outputs"=w516:dbl[], "Sweep Parameters"=w512:sgl[], "Start Sweep"=w507:bool, "Manual Cmd"=w506:bool)
        n223 = Index Array(array=w515) -> (element #1=w521:bool, element #2=w520:bool, element #3=w519:bool, element #4=w518:bool)  [unwired: 4 in]
        n224 = Index Array(array=w516) -> (element #1=w517:dbl, element #2=w514:dbl, element #3=w513:dbl)  [unwired: 3 in]
        n225 = Index Array(array=w512) -> (element #1=w511:sgl, element #2=w510:sgl, element #3=w509:sgl, element #4=w508:sgl)  [unwired: 4 in]
        n226 = case shown="False" w501 {
          tunnel: w504 -> [w572 w588]
          tunnel: [w571 w587] -> w522
          tunnel: "10kHz Loop Control (us)" -> [w570 w586]
          tunnel: "AI Loop Control (us)" -> [w569 w585]
          tunnel: w521 -> [w568 w584]
          tunnel: w520 -> [w567 w583]
          tunnel: w519 -> [w566 w582]
          tunnel: w518 -> [w565 w581]
          tunnel: w517 -> [w564 _]
          tunnel: w514 -> [w563 w580]
          tunnel: w513 -> [w562 w579]
          tunnel: w511 -> [w561 w578]
          tunnel: w510 -> [w560 w577]
          tunnel: w509 -> [w559 w576]
          tunnel: w508 -> [w558 w575]
          tunnel: w507 -> [w557 w574]
          tunnel: w506 -> [w556 w573]
          frame False {
            # "Write everything"
            n227 = xnode "Read/Write Control"("FPGA VI Reference In"=w572, "10kHz Loop Control (us)"=w570, "AI Loop Control (us)"=w569, "RMC/DO0"=w568, "RMC/DO1"=w567, "RMC/DO2"=w566, "RMC/DO3"=w565, "Position Command"=w564, "PS Command"=w563, "AO3 Spare"=w562, "Total Samples"=w561, "End Ht Cmd"=w560, "Start Ht Cmd"=w559, "Sweep Count"=w558, "Start Sweep"=w557, "Manual Cmd"=w556) -> ("FPGA VI Reference Out"=w571:refnum<k20>)  [unwired: 1 in, 1 out]
          }
          frame True {
            # "Prevent height movement"
            n228 = xnode "Read/Write Control"("FPGA VI Reference In"=w588, "10kHz Loop Control (us)"=w586, "AI Loop Control (us)"=w585, "RMC/DO0"=w584, "RMC/DO1"=w583, "RMC/DO2"=w582, "RMC/DO3"=w581, "PS Command"=w580, "AO3 Spare"=w579, "Total Samples"=w578, "End Ht Cmd"=w577, "Start Ht Cmd"=w576, "Sweep Count"=w575, "Start Sweep"=w574, "Manual Cmd"=w573) -> ("FPGA VI Reference Out"=w587:refnum<k20>)  [unwired: 1 in, 1 out]
          }
        }
      }
      frame "Handle Sweep Start" {
        n229 = Wait (ms)(milliseconds to wait=u32 1) -> ()  [unwired: 1 out]
        n230 = Insert Into Array(array=w590, index=0, new element="Write Outputs" ("new element/subarray")) -> (w589:string[])
        n231 = Bundle By Name(cluster=w595, "Start Sweep"=FALSE) -> (w594:T2)
      }
    }
  }
  n232 = flat-sequence {
    tunnel: w10 -> [w598]
    frame #0 {
      n233 = Wait on Occurrence(2:w598) -> ()  [unwired: 2 in, 1 out]
    }
    frame #1 {
      n234 = call "AI RT FIFO.vi"("Mode"=Stream_RT_FIFO_Mode."Create", "Buffer Size"=800, "# of elements"=8) -> ()  [unwired: 10 in, 3 out]
    }
    frame #2 {
      n235 = control-ref of="Stream Stop"() -> (w604:refnum<vi>)
      n236 = property class="Bool (strict)"(reference=w604, "Value"=FALSE) -> (reference out=w602:refnum<vi>)  [unwired: 1 in, 1 out]
      n237 = call "Loop (Data Stream).vi"("Stop"=w602) -> ()  [unwired: 10 in, 1 out]
    }
    frame #3 {
      n238 = call "AI RT FIFO.vi"("Mode"=Stream_RT_FIFO_Mode."Delete") -> ()  [unwired: 12 in, 3 out]
    }
  }
  n239 = call "RT Engine.vi"("Error In"=w16) -> ()  [unwired: 11 in]
  n240 = while {
    tunnel: w16 -> [w608]
    stop <- FALSE stop-if-true
    n241 = call <vilib>:"RT Get CPU Loads.vi"("error in (no error)"=w608) -> ("CPU loads"=w611:T9[])  [unwired: 9 in, 1 out]
    n242 = Index Array(array=w611) -> (element=w610:T9)  [unwired: 1 in]
    n243 = Unbundle By Name(w610) -> ("Total (%)"=→"Total (%)":dbl)
    n244 = Wait (ms)(milliseconds to wait=u32 500) -> ()  [unwired: 1 out]
  }
  n245 = Destroy Stream Endpoint(11:w2) -> ()  [unwired: 1 in, 1 out]
